vi "Initialize AI Task.vi"(8 "error in (no error)":errorcluster, 11 "BNT_DAQmx-MCSV-AIAvg in":refnum<class "BNT_DAQmx-MCSV-AIAvg.lvclass">) -> (0 "error out":errorcluster, 3 "AI DAQmx Task":refnum<k21>)   [LabVIEW 2018, in "BNT_DAQmx.lvlib" / "BNT_DAQmx-MCSV-AIAvg.lvclass"]
doc: "Initialize DAQmx Analog Input task.\n\n<b>Default Implementation:</b> Analog Input Voltage\n\nThis dynamic dispatch VI can be overritten by derived classes to implement other analog input tasks."
uses:
  BNT_DAQmx-MCSV-AIAvg.lvclass
  BNT_DAQmx-MCSV-AIAvg.lvclass/BNT_DAQmx-MCSV-AIAvg.ctl
  <vilib>/DAQmx/configure/timing.llb/DAQmx Timing (Sample Clock).vi
  BNT_DAQmx-MCSV/BNT_DAQmx-MCSV.lvclass
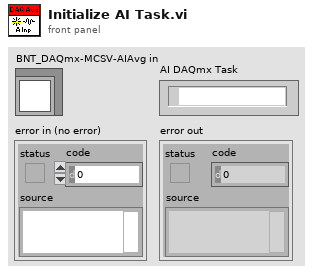
[diagram p1: front panel]
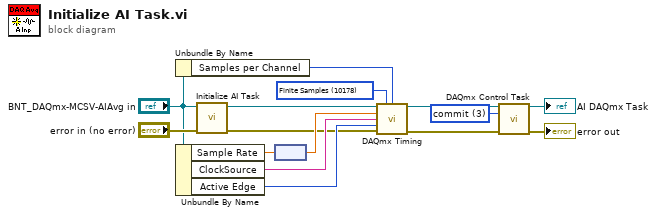
[diagram p0: block diagram]
diagram:
  w5 = 3 items=["verify"=2, "reserve"=4, "commit"=3, "unreserve"=5, "abort"=6] ("action")
  w14 = 10178 items=["Finite Samples"=10178, "Continuous Samples"=10123, "Hardware Timed Single Point"=12522] ("sample mode")
  n1 = Unbundle By Name("BNT_DAQmx-MCSV-AIAvg in") -> ("Samples per Channel"=w12:i32)
  n2 = Unbundle By Name("BNT_DAQmx-MCSV-AIAvg in") -> ("Sample Rate"=w9:dbl[unit], "ClockSource"=w8:tag, "Active Edge"=w7:i32)
  n3 = call-parent "Initialize AI Task.vi"("error in (no error)"="error in (no error)", "BNT_DAQmx-MCSV in"="BNT_DAQmx-MCSV-AIAvg in") -> ("error out"=w1:errorcluster, "AI DAQmx Task"=w2:refnum<k21>)  [unwired: 8 in]
  n4 = node(w9) -> (w13:dbl)
  n5 = call-poly <vilib>:"DAQmx Timing.vi"("task/channels in"=w2, "sample mode"=w14, "samples per channel"=w12, "rate"=w13, "source"=w8, "active edge"=w7, "error in"=w1) -> ("task out"=w15:refnum<k21>, "error out"=w4:errorcluster)  [unwired: 7 in]
  n6 = call <vilib>:"DAQmx Control Task.vi"("task/channels in"=w15, "action"=w5, "error in"=w4) -> ("task out"=→"AI DAQmx Task":refnum<k21>, "error out"=→"error out":errorcluster)  [unwired: 11 in]
